vi "libssh2_channel_forward_cancel.vi"(8 "error in (no error)":errorcluster, 11 "listener":T1) -> (0 "error out":errorcluster, 3 "return value":i32)   [LabVIEW 2013, in "libssh2.lvlib"]
doc: "Instructs the remote host to stop listening for new connections on a previously requested port."
uses:
  libssh2.lvlib
  Listener Refnum.ctl
  Global Settings.vi
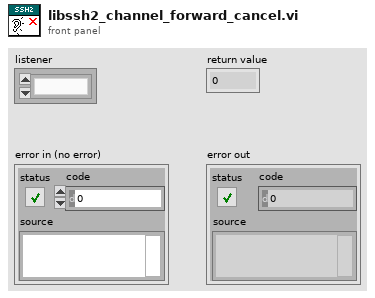
[diagram p1: front panel]
types:
  T1 = typedef "libssh2.lvlib/Listener Refnum.ctl" = refnum<k1>
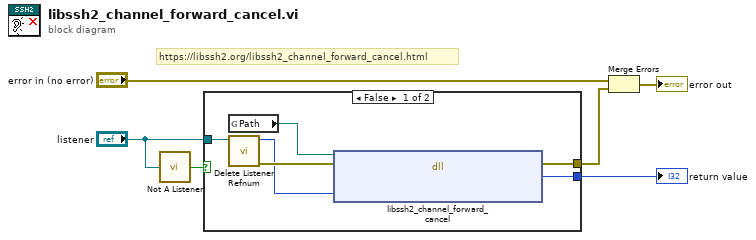
[diagram p0: block diagram]
diagram:
  # "https://libssh2.org/libssh2_channel_forward_cancel.html"
  n1 = call "Not A Listener.vi"("listener"="listener") -> ("Not a Listener?"=w1:bool)
  n2 = case shown="False" w1 {
    tunnel: [w12 _] -> w6
    tunnel: "listener" -> [w10 _]
    tunnel: [w8 _] -> w3
    frame False {
      n3 = global read "Global Settings.vi" "Path"() -> (w7:path)
      n4 = call "Delete Listener Refnum.vi"("listener"=w10) -> ("error out"=w11:errorcluster, "LIBSSH2_LISTENER*"=w9:u64)  [unwired: 9 in]
      n5 = dll-call lib="C:/Users/pasca/source/repos/libssh2-labview/libssh2/libssh2**.*" fn="libssh2_channel_forward_cancel"(path in=w7, error in=w11, "listener"=w9) -> (error out=w8:errorcluster, "return value"=w12:i32)  [unwired: 2 in, 1 out]
    }
    frame True {
    }
  }
  "return value" <- w6
  n6 = Merge Errors("error in (no error)", w3) -> (→"error out":errorcluster)
